vi "Open File.vi"(7 "file mode":T1=enum."create/replace", 8 "error in (no error)":errorcluster, 11 "Shared Memory in":refnum<class "Shared Memory.lvclass">) -> (0 "error out":errorcluster, 3 "Shared Memory out":refnum<class "Shared Memory.lvclass">)   [LabVIEW 2013, in "Linux RT IPC.lvlib" / "Shared Memory.lvlib" / "Shared Memory.lvclass"]
uses:
  Shared Memory.lvclass
  Public/Controls/file mode.ctl
  Shared Memory.lvclass/Shared Memory.ctl
  Shared Memory.lvlib
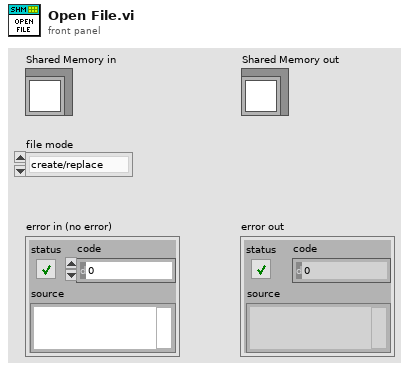
[diagram p1: front panel]
types:
  T1 = typedef "Linux RT IPC.lvlib/Shared Memory.lvlib/file mode.ctl" = enum16{"open", "create/replace"}
  T2 = cluster{"create":bool, "excl":bool, "truncate":bool}
  T3 = cluster{"owner":cluster{"read":bool, "write":bool, "execute":bool}, "group":cluster{"read":bool, "write":bool, "execute":bool}, "everyone":cluster{"read":bool, "write":bool, "execute":bool}}
  T4 = typedef "Linux RT IPC.lvlib/Shared Memory.lvlib/Shared Memory.lvclass/mode_t.ctl" = u32
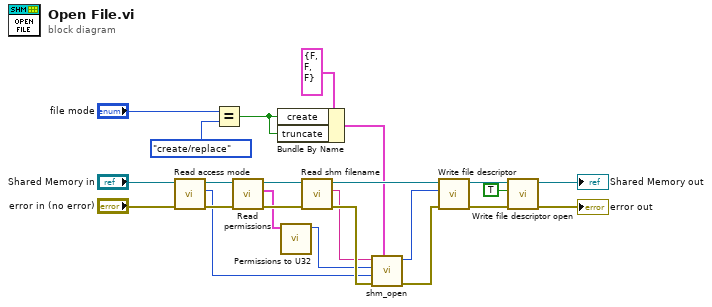
[diagram p0: block diagram]
diagram:
  n1 = call "Read access mode.vi"("error in (no error)"="error in (no error)", "Shared Memory in"="Shared Memory in") -> ("error out"=w14:errorcluster, "access mode"=w12:enum16{"read only", "read and write"}, "Shared Memory out"=w13:refnum<class "Shared Memory.lvclass">)  [unwired: 7 in]
  n2 = Equal?(x="file mode", y=file_mode."create/replace") -> (x = y?=w20:bool)
  n3 = call "Read permissions.vi"("error in (no error)"=w14, "Shared Memory in"=w13) -> ("error out"=w10:errorcluster, "permissions"=w9:T3, "Shared Memory out"=w11:refnum<class "Shared Memory.lvclass">)  [unwired: 7 in]
  n4 = Bundle By Name(cluster=T2 {"create"=FALSE, "excl"=FALSE, "truncate"=FALSE} ("flags"), "create"=w20, "truncate"=w20) -> (w1:T2)
  n5 = call "Permissions to U32.vi"("permissions"=w9) -> ("packed permissions"=w15:T4)  [unwired: 10 in]
  n6 = call "Read shm filename.vi"("error in (no error)"=w10, "Shared Memory in"=w11) -> ("error out"=w24:errorcluster, "shm filename"=w8:string, "Shared Memory out"=w6:refnum<class "Shared Memory.lvclass">)  [unwired: 7 in]
  n7 = call "shm_open.vi"("flags"=w1, "error in (no error)"=w24, "access mode (read/write)"=w12, "permissions (0777)"=w15, "shared memory name"=w8) -> ("error out"=w7:errorcluster, "file descriptor"=w5:i32)  [unwired: 5 in]
  n8 = call "Write file descriptor.vi"("error in (no error)"=w7, "file descriptor"=w5, "Shared Memory in"=w6) -> ("error out"=w19:errorcluster, "Shared Memory out"=w18:refnum<class "Shared Memory.lvclass">)  [unwired: 7 in]
  n9 = call "Write file descriptor open.vi"("error in (no error)"=w19, "file descriptor open"=TRUE, "Shared Memory in"=w18) -> ("error out"=→"error out":errorcluster, "Shared Memory out"=→"Shared Memory out":refnum<class "Shared Memory.lvclass">)  [unwired: 7 in]
